vi "cornell-K0sh.vi"(6 "Numeric":i32=500, 8 "τ":dbl=1.0, 9 "h":dbl, 10 "s":dbl, 11 "ω":dbl) -> (0 "Ks(ω)":cdb)   [LabVIEW 2020]
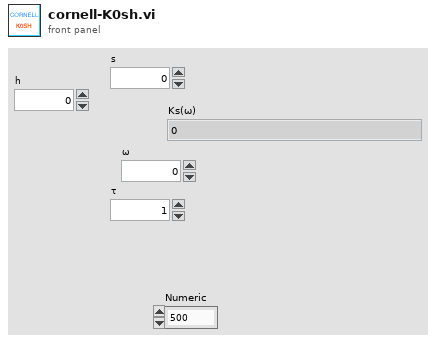
[diagram p1: front panel]
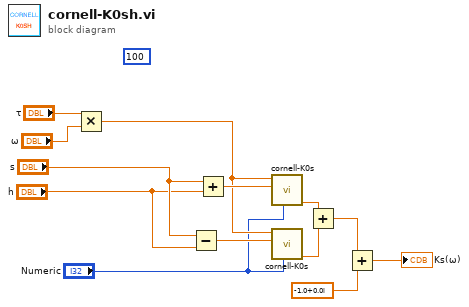
[diagram p0: block diagram]
diagram:
  (unwired) 100
  n1 = Multiply(x="τ", y="ω") -> (x*y=w2:dbl)
  n2 = Subtract(x="s", y="h") -> (x-y=w10:dbl)
  n3 = Add(x="s", y="h") -> (x+y=w11:dbl)
  n4 = call "cornell-K0s.vi"("Numeric"="Numeric", "s"=w11, "ω"=w2) -> ("Ks(ω)"=w9:cdb)  [unwired: 8 in]
  n5 = call "cornell-K0s.vi"("Numeric"="Numeric", "s"=w10, "ω"=w2) -> ("Ks(ω)"=w8:cdb)  [unwired: 8 in]
  n6 = Add(x=w9, y=w8) -> (x+y=w7:cdb)
  n7 = Add(x=w7, y=cdb -1.0+0.0i ("x")) -> (x+y=→"Ks(ω)":cdb)
